vi "Intake deal with joysticks.vi"(1 "Index % output":dbl, 2 "Negative Throttle (%)":dbl, 3 "Extend?":bool, 4 "Positive Throttle (%)":dbl) -> (0 "Intake Teleop Command":T1)   [LabVIEW 2019]
uses:
  Intake Command Type Def.ctl
  Intake Mode Type Def.ctl
  <vilib>/Rock Robotics/WPI/Solenoid/WPI_SolenoidValue.ctl
panel:
  # "INTAKE AUTO-EXTENDS / RETRACTS IF TRIGGERS PRESSED >75%\nOtherwise stays at prior state"
  # "Positive is IN\nNEGATIVE IS OUT"
  # "So that when index runs, intake also will"
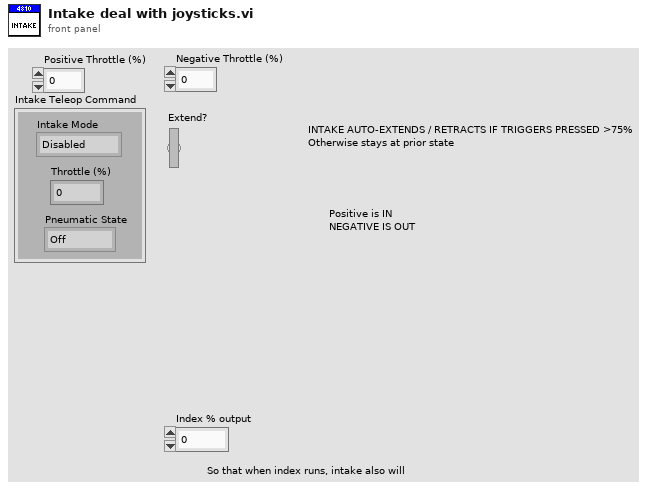
[diagram p1: front panel]
types:
  T1 = typedef "Intake Command Type Def.ctl" = cluster{"Intake Mode":T2, "Throttle (%)":dbl, "Pneumatic State":T3}
  T2 = typedef "Intake Mode Type Def.ctl" = enum16{"Disabled", "Enabled"}
  T3 = typedef "WPI_SolenoidValue.ctl" = enum16{"Off", "On", "Forward", "Reverse"}
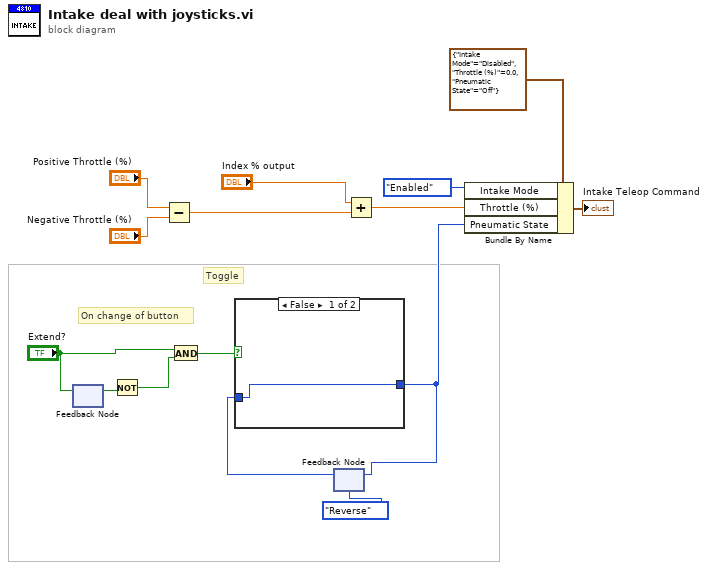
[diagram p0: block diagram]
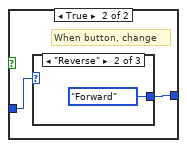
[diagram p2: hidden frame]
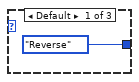
[diagram p3: hidden frame]
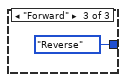
[diagram p4: hidden frame]
diagram:
  # "Toggle"
  # "On change of button"
  n1 = feedback-in #1("Extend?") -> ()
  n2 = feedback #1() -> (w7:bool)  [unwired: 1 in]
  n3 = Not(x=w7) -> (.not. x?=w5:bool)
  n4 = Subtract(x="Positive Throttle (%)", y="Negative Throttle (%)") -> (x-y=w3:dbl)
  n5 = And(x="Extend?", y=w5) -> (x .and. y?=w4:bool)
  n6 = feedback #2(WPI_SolenoidValue."Reverse" ("Pneumatic State")) -> (w9:T3)
  n7 = case shown="False" w4 {
    tunnel: [w16 w18] -> w8
    tunnel: w9 -> [w16 w17]
    frame False {
    }
    frame True {
      # "When button, change"
      n8 = case shown="\"Reverse\"" w17 {
        tunnel: [WPI_SolenoidValue."Reverse" ("Pneumatic State") WPI_SolenoidValue."Forward" ("Pneumatic State") WPI_SolenoidValue."Reverse" ("Pneumatic State")] -> w18
        frame Default {
        }
        frame "Reverse" {
        }
        frame "Forward" {
        }
      }
    }
  }
  n9 = feedback-in #2(w8) -> ()
  n10 = Add(x="Index % output", y=w3) -> (x+y=w1:dbl)
  n11 = Bundle By Name(cluster=T1 {"Intake Mode"=enum."Disabled", "Throttle (%)"=0.0, "Pneumatic State"=enum."Off"} ("Teleop Intake Command"), "Intake Mode"=Intake_Mode_Type_Def."Enabled", "Throttle (%)"=w1, "Pneumatic State"=w8) -> (→"Intake Teleop Command":T1)
